vi "Choreo_ReadTrajectoryFile_FGV_Example.vi"() -> ()   [LabVIEW 2019]
uses:
  <vilib>/Rock Robotics/WPI/ThirdParty/ChoreoLib/ChoreoLib.lvlib
panel:
  out "error out":errorcluster
  # "Read Trajectory JSON File and Write to Functional Global Variable"
  # "See block diagram"
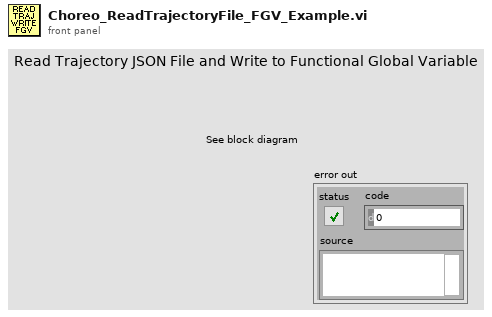
[diagram p1: front panel]
types:
  T1 = typedef "ChoreoLib.lvlib/ChoreoTrajectorySwerve.ctl" = cluster{"name":string, "samples":T2[], "splits":i32[], "events":T3[]}
  T2 = typedef "ChoreoLib.lvlib/ChoreoSwerveSample.ctl" = cluster{"timestamp":dbl, "x":dbl, "y":dbl, "heading":dbl, "velocityX":dbl, "velocityY":dbl, "angularVelocity":dbl, "accelX":dbl, "accelY":dbl, "accelAngular":dbl, "forceX":dbl[], "forceY":dbl[]}
  T3 = typedef "ChoreoLib.lvlib/ChoreoEventMarker.ctl" = cluster{"TimeStamp":dbl, "Name":string}
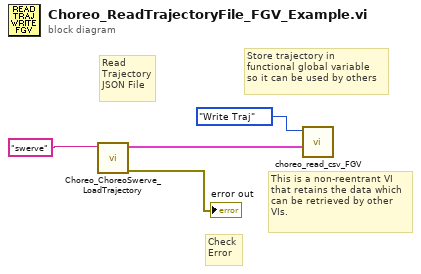
[diagram p0: block diagram]
diagram:
  # "Check\nError"
  # "This is a non-reentrant VI\nthat retains the data which\ncan be retrieved by other\nVIs."
  # "Read\nTrajectory\nJSON File"
  # "Store trajectory in\nfunctional global variable\nso it can be used by others"
  n1 = call <vilib>:"Choreo_ChoreoSwerve_LoadTrajectory.vi"("FileName"="swerve" ("CSV File Name")) -> ("error out"=→"error out":errorcluster, "ChoreoTrajectorySwerve"=w1:T1)  [unwired: 8 in, 1 out]
  n2 = call "choreo_read_csv_FGV.vi"("inTRAJECTORY"=w1, "Command"=enum16{"Read Traj", "Write Traj"}."Write Traj") -> ()  [unwired: 9 in, 1 out]
